vi "Test PQ modes.vi"() -> ()   [LabVIEW 2016]
uses:
  <vilib>/JDP Science/PostgreSQL Library/Connection/PQ Connection.lvclass
panel:
  in  "path":path
  out "Results":cluster{"Array":i32[], dbl[]}[](graph)
  in  "Method":T1(ring)
  in  "Array":i32[](array[numeric])
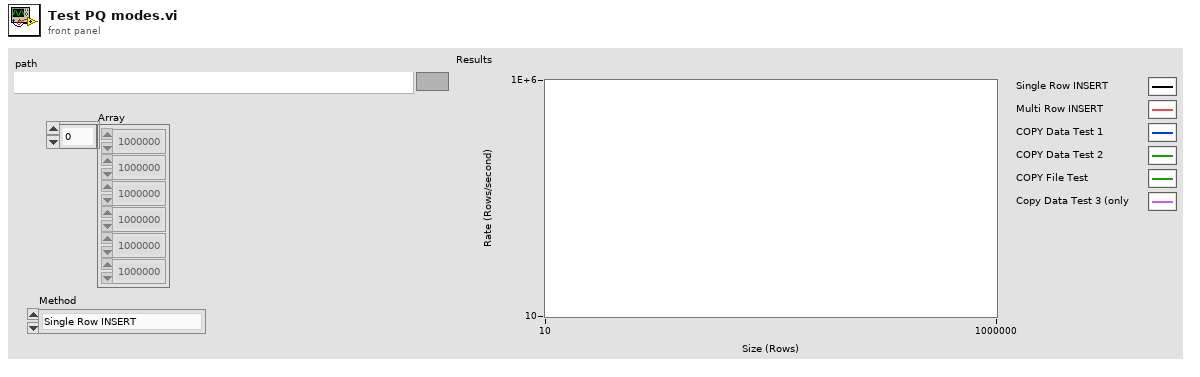
[diagram p1: front panel]
types:
  T1 = enum16{"Single Row INSERT", "Multi Row INSERT", "COPY", "COPY file"}
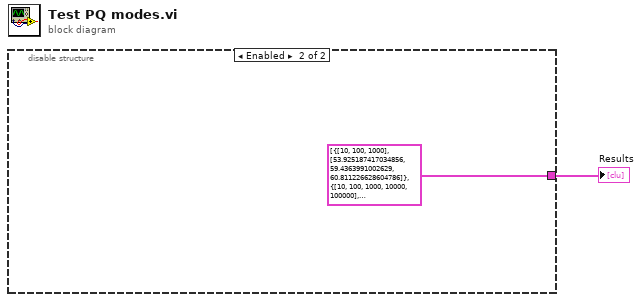
[diagram p0: block diagram]
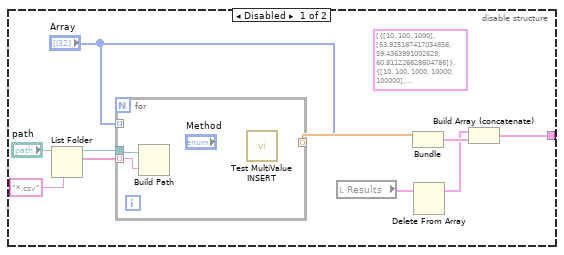
[diagram p2: hidden frame]
diagram:
  n1 = disable-structure shown="Enabled" {
    disable-tunnel: [w9 cluster{"Array":i32[], dbl[]}[] [{"Array"=[10, 100, 1000], [53.925187417034856, 59.4363991002629, 60.811226628604786]}, {"Array"=[10, 100, 1000, 10000, 100000], [283.65414626003354, 2440.774605580749, 6544.806724206658, 10753.910418198006, 17465.95810482594]}, {"Array"=[10, 100, 1000, 10000, 100000], [192.36836226792013, 1766.1946793800532, 7328.5253313695175, 10846.864617124398, 13535.967122045666]}, {"Array"=[10, 100, 1000, 10000, 100000, 1000000], [195.24690923493955, 1768.6061817798723, 7307.238689810668, 11150.768198951346, 13422.74077801498, 13323.240428011148]}] ("XY Graph")] -> w1
    frame Disabled {
      (unwired) cluster{"Array":i32[], dbl[]}[] [{"Array"=[10, 100, 1000], [53.925187417034856, 59.4363991002629, 60.811226628604786]}, {"Array"=[10, 100, 1000, 10000, 100000], [283.65414626003354, 2440.774605580749, 6544.806724206658, 10753.910418198006, 17465.95810482594]}, {"Array"=[10, 100, 1000, 10000, 100000], [192.36836226792013, 1766.1946793800532, 7328.5253313695175, 10846.864617124398, 13535.967122045666]}, {"Array"=[10, 100, 1000, 10000, 100000, 1000000], [195.24690923493955, 1768.6061817798723, 7307.238689810668, 11150.768198951346, 13422.74077801498, 13323.240428011148]}] ("XY Graph")
      n2 = List Folder(path="path", pattern="*.csv") -> (path out=w6:path, filenames=w5:string[])  [unwired: 2 in, 2 out]
      n3 = for {
        tunnel: [_] -> w11 mode=indexing
        tunnel: w6 -> [w14]
        tunnel: w5 -> [w13] mode=indexing
        tunnel: "Array" -> [w12] mode=indexing
        n4 = Build Path(base path=w14, name or relative path=w13) -> ()  [unwired: 1 out]
        n5 = call "Test MultiValue INSERT.vi"() -> ()  [unwired: 12 in]
      }
      n6 = local read "Results"() -> (w3:cluster{"Array":i32[], dbl[]}[])
      n7 = Bundle("Array"="Array", w11) -> (w10:cluster{"Array":i32[], void})  [unwired: 1 in]
      n8 = Delete From Array(array=w3) -> (array with subset deleted=w2:cluster{"Array":i32[], dbl[]}[])  [unwired: 2 in, 1 out]
      n9 = Build Array (concatenate)(w2, w10) -> (w9:cluster{"Array":i32[], dbl[]}[])
    }
    frame Enabled {
    }
  }
  "Results" <- w1
